vi "DK240 ErrHandler.vi"(6 "error in":errorcluster) -> (0 "error out":errorcluster)   [LabVIEW 2010]
doc: "Ce VI prend en charge la gestions des erreurs. Il décode les code d'erreurs du monochromateur et affiche un message de description."
uses:
  <vilib>/Utility/error.llb/DialogType.ctl
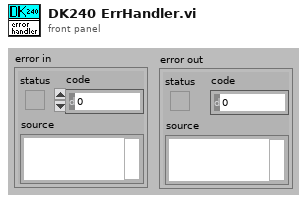
[diagram p1: front panel]
types:
  T1 = typedef "DialogType.ctl" = u16
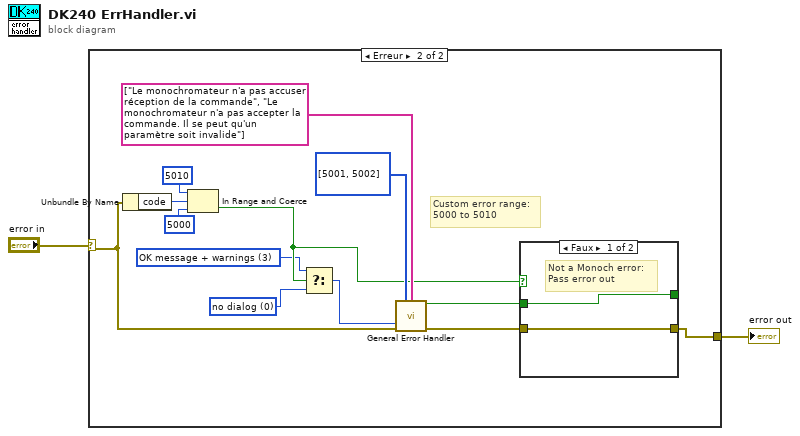
[diagram p0: block diagram]
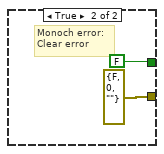
[diagram p3: hidden frame]
diagram:
  n1 = case shown="Erreur" "error in" {
    selector: "error in" -> [w3 w9]
    tunnel: [w3 w11] -> w1
    frame No Error {
    }
    frame Error {
      w6 = T1 3 items=["no dialog", "OK message", "continue or stop message", "OK message + warnings", "continue/stop + warnings"] ("type of dialog (OK msg:1)")
      w5 = T1 0 items=["no dialog", "OK message", "continue or stop message", "OK message + warnings", "continue/stop + warnings"] ("type of dialog (OK msg:1)")
      # "Custom error range:\n5000 to 5010"
      n2 = Unbundle By Name(w9) -> ("code"=w8:i32)
      n3 = In Range and Coerce(upper limit=5010, x=w8, lower limit=5000) -> (In Range?=w7:bool)  [unwired: 1 out]
      n4 = Select(t=w6, s=w7, f=w5) -> (s? t:f=w4:T1)
      n5 = call <vilib>:"General Error Handler.vi"("[user-defined codes]"=i32[] [5001, 5002], "[user-defined descriptions]"=string[] ["Le monochromateur n'a pas accuser réception de la commande", "Le monochromateur n'a pas accepter la commande. Il se peut qu'un paramètre soit invalide"], "type of dialog (OK msg:1)"=w4, "error in (no error)"=w9) -> ("error?"=w13:bool, "error out"=w16:errorcluster)  [unwired: 7 in, 3 out]
      n6 = case shown="Faux" w7 {
        tunnel: [w18 errorcluster {"status"=FALSE, "code"=0, "source"=""} ("error out")] -> w11
        tunnel: w16 -> [w18 _]
        tunnel: [w17 FALSE ("error?")] -> _
        tunnel: w13 -> [w17 _]
        frame False {
          # "Not a Monoch error:\nPass error out"
        }
        frame True {
          # "Monoch error:\nClear error"
        }
      }
    }
  }
  "error out" <- w1
